vi "Arithmetic Calculator.vi"() -> ()   [LabVIEW 2016]
panel:
  out "Loops":i32
  in  "stop":bool
  out "x/y":dbl
  out "x-y":dbl
  out "x*y":dbl
  out "x+y":dbl
  in  "Numeric 2":dbl
  in  "Numeric":dbl
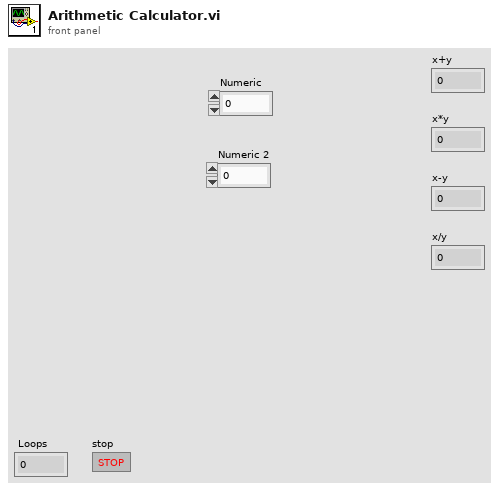
[diagram p1: front panel]
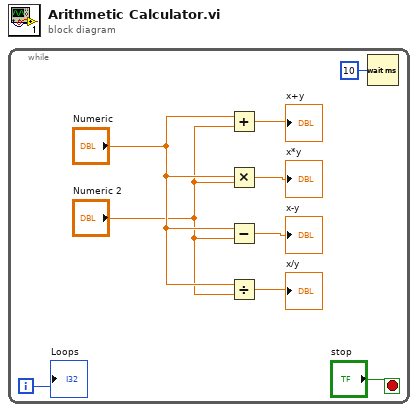
[diagram p0: block diagram]
diagram:
  n1 = while {
    i -> [w2]
    stop <- "stop" stop-if-true
    n2 = Add(x="Numeric", y="Numeric 2") -> (x+y=→"x+y":dbl)
    n3 = Multiply(x="Numeric", y="Numeric 2") -> (x*y=→"x*y":dbl)
    n4 = Subtract(x="Numeric", y="Numeric 2") -> (x-y=→"x-y":dbl)
    n5 = Divide(x="Numeric", y="Numeric 2") -> (x/y=→"x/y":dbl)
    n6 = Wait (ms)(milliseconds to wait=u32 10) -> ()  [unwired: 1 out]
    "Loops" <- w2
  }
